vi "Parse Response Data.vi"(8 "error in":errorcluster, 11 "EF20 in":refnum<class "EF20.lvclass">) -> (0 "error out":errorcluster, 3 "EF20 out":refnum<class "EF20.lvclass">)   [LabVIEW 2018, in "EF20.lvlib" / "EF20.lvclass"]
uses:
  EF20.lvclass
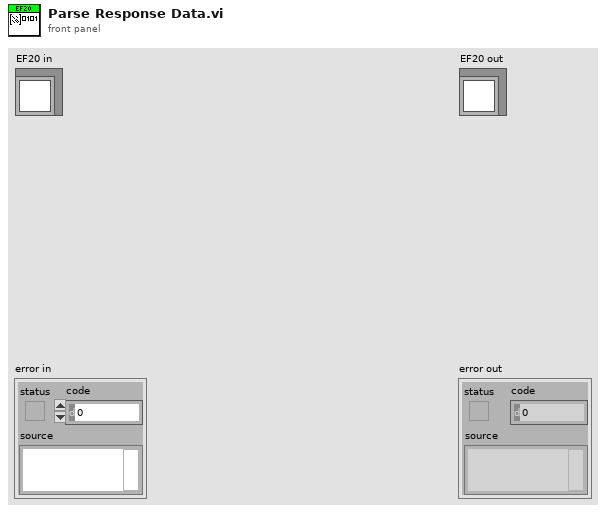
[diagram p1: front panel]
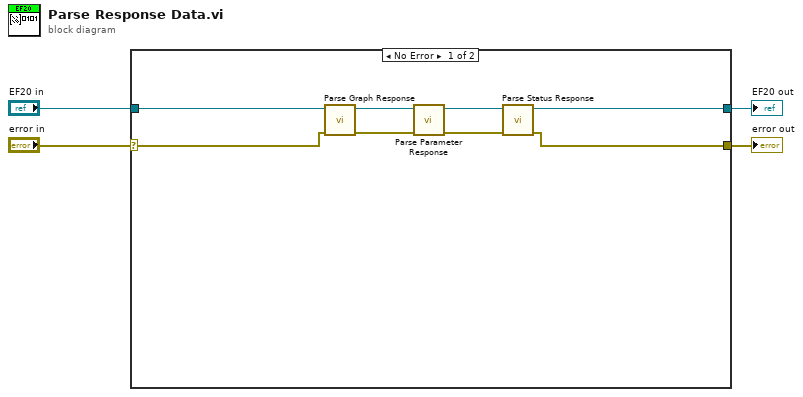
[diagram p0: block diagram]
diagram:
  n1 = case shown="No Error" "error in" {
    selector: "error in" -> [w6 w14]
    tunnel: [w5 w14] -> w3
    tunnel: [w9 w13] -> w1
    tunnel: "EF20 in" -> [w10 w13]
    frame No Error {
      n2 = call "Parse Graph Response.vi"("error in"=w6, "EF20 in"=w10) -> ("error out"=w8:errorcluster, "EF20 out"=w12:refnum<class "EF20.lvclass">)  [unwired: 8 in]
      n3 = call "Parse Parameter Response.vi"("error in"=w8, "EF20 in"=w12) -> ("error out"=w7:errorcluster, "EF20 out"=w11:refnum<class "EF20.lvclass">)  [unwired: 8 in]
      n4 = call "Parse Status Response.vi"("error in"=w7, "EF20 in"=w11) -> ("error out"=w5:errorcluster, "EF20 out"=w9:refnum<class "EF20.lvclass">)  [unwired: 8 in]
    }
    frame Error {
    }
  }
  "error out" <- w3
  "EF20 out" <- w1
